vi "InitAction.vi"(6 "InstrumentName":string, 7 "VisaRessIn":refnum<visa-resource-name>, 8 "error in (no error)":errorcluster caption="entrée d'erreur (pas d'erreur)", 9 "FirstClassInst":bool, 10 "Function":string, 11 "Device en entrée":refnum<class "BaseDevice.lvclass"> caption="DNL_LabVIEW Object in") -> (0 "error out":errorcluster caption="sortie d'erreur", 3 "Device en sortie":refnum<class "BaseDevice.lvclass"> caption="DNL_LabVIEW Object out")   [LabVIEW 2019, in "BaseDevice.lvclass"]
uses:
  BaseDevice.lvclass
  BaseDevice_Func.ctl
panel:
  out "VisaRessOut":refnum<visa-resource-name>
  in  "Dev_Func":T1
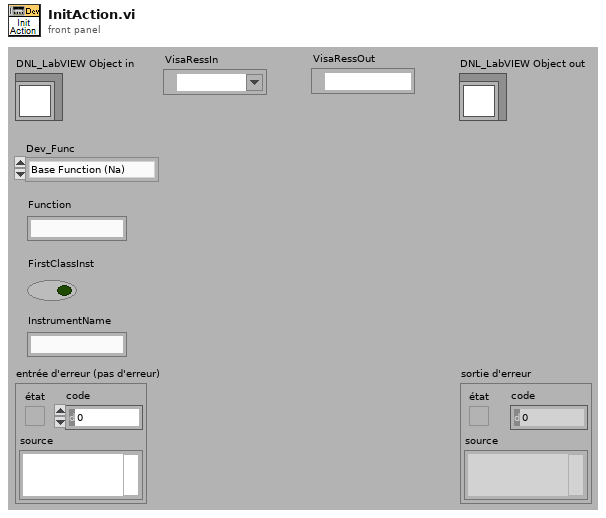
[diagram p1: front panel]
types:
  T1 = typedef "BaseDevice.lvclass/BaseDevice_Func.ctl" = enum16{"Base Function (Na)"}
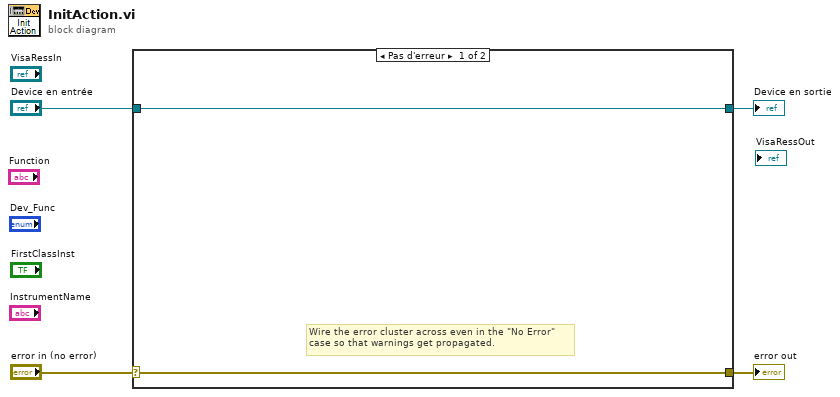
[diagram p0: block diagram]
diagram:
  n1 = case shown="Pas d'erreur" "error in (no error)" {
    selector: "error in (no error)" -> [w6 w8]
    tunnel: [w6 w8] -> w3
    tunnel: [w5 w7] -> w1
    tunnel: "Device en entrée" -> [w5 w7]
    frame No Error {
      # "Wire the error cluster across even in the \"No Error\"\ncase so that warnings get propagated."
    }
    frame Error {
    }
  }
  "error out" <- w3
  "Device en sortie" <- w1
